vi "write servers jsons.vi"(8 "error in (no error)":errorcluster, 11 "Save Image in":refnum<class "Save Image.lvclass">) -> (0 "error out":errorcluster, 3 "Save Image out":refnum<class "Save Image.lvclass">)   [LabVIEW 2018, in "Save Image.lvclass"]
uses:
  Save Image.lvclass
  Save Image.lvclass/Save Image.ctl
  Channel/Channel.lvclass/Channel.ctl
  Server/Server.lvclass/Server.ctl
  State Machine/State Machine.lvclass
  RxTx/RxTx.lvclass
  Simulated_CCD_Camera/Simulated Camera.lvclass
  Log File/Log File.lvclass
  Error log/Error log.lvclass
  Keywords Log File/Keywords Log File.lvclass
  Server/Server.lvclass
  Channel/Channel.lvclass
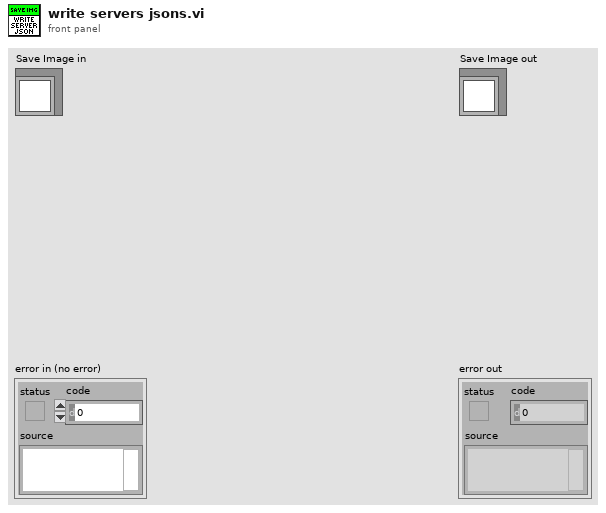
[diagram p1: front panel]
types:
  T1 = cluster{"State Machine.lvclass":refnum<class "State Machine.lvclass">, "RxTx.lvclass":refnum<class "RxTx.lvclass">, "Simulated_CCD_Camera.lvclass":refnum<class "Simulated Camera.lvclass">, "Save_Header_RxTx.lvclass":refnum<class "RxTx.lvclass">, "Status SM.lvclass":refnum<class "State Machine.lvclass">, "Status RxTx.lvclass":refnum<class "RxTx.lvclass">, "Log File.lvclass":refnum<class "Log File.lvclass">, "Error log.lvclass":refnum<class "Error log.lvclass">, "Keywords Log File.lvclass":refnum<class "Keywords Log File.lvclass">, "servers array":refnum<class "Server.lvclass">[]}
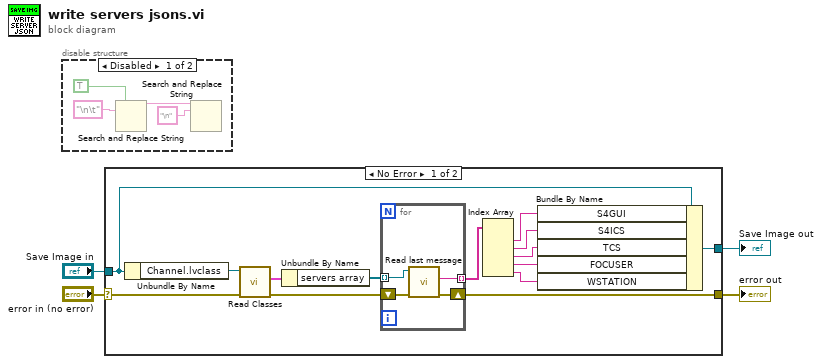
[diagram p0: block diagram]
diagram:
  n1 = disable-structure "Diagram Disable Structure" shown="Disabled" {
    frame Disabled {
      n2 = Search and Replace String(replace all?=TRUE ("replace all? (F)"), search string="\n\t") -> (result string=w8:string)  [unwired: 6 in, 3 out]
      n3 = Search and Replace String(input string=w8, search string="\n") -> ()  [unwired: 6 in, 4 out]
    }
    frame Enabled {
    }
  }
  n4 = case shown="No Error" "error in (no error)" {
    selector: "error in (no error)" -> [w20 w28]
    tunnel: [w18 w28] -> w3
    tunnel: [w16 w27] -> w1
    tunnel: "Save Image in" -> [w17 w27]
    frame No Error {
      n5 = Unbundle By Name(w17) -> ("Channel.lvclass"=w21:refnum<class "Channel.lvclass">)
      n6 = call "Read Classes.vi"("error in (no error)"=w20, "Channel in"=w21) -> ("error out"=w19:errorcluster, "Classes"=w22:T1)  [unwired: 7 in, 1 out]
      n7 = Unbundle By Name(w22) -> ("servers array"=w9:refnum<class "Server.lvclass">[])
      n8 = for {
        tunnel: w9 -> [w26] mode=indexing
        tunnel: [w25] -> w15 mode=indexing
        shift-right: [w23] -> w18
        shift-left: w19 -> [w24]
        n9 = call "Read last message.vi"("error in (no error)"=w24, "Server in"=w26) -> ("error out"=w23:errorcluster, "last message"=w25:string)  [unwired: 7 in, 1 out]
      }
      n10 = Index Array(array=w15) -> (element #1=w14:string, element #2=w10:string, element #3=w13:string, element #4=w12:string, element #5=w11:string)  [unwired: 5 in]
      n11 = Bundle By Name(cluster=w17, "S4GUI"=w14, "S4ICS"=w10, "TCS"=w13, "FOCUSER"=w12, "WSTATION"=w11) -> (w16:refnum<class "Save Image.lvclass">)
    }
    frame Error {
    }
  }
  "error out" <- w3
  "Save Image out" <- w1
